vi "S2C_InitTest.vi"(8 "Error In":errorcluster, 11 "TestName":string) -> (0 "Error Out":errorcluster)   [LabVIEW 2015]
doc: "Detects an error and calls the error case to process the error."
uses:
  XML/S2C_XML_Globals.vi
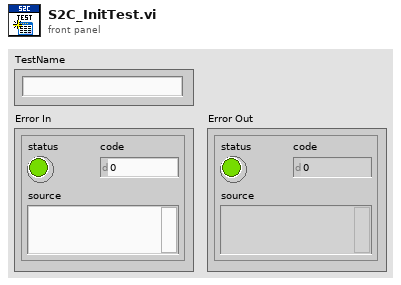
[diagram p1: front panel]
types:
  T1 = cluster{"TestName":string, "TestDateTime":string, "TestStatus":string, "Comment":string}
  T2 = cluster{"TestName":string, "TestDateTime":string, "TestStatus":string, "TestClientID":string, "IS_TestID":string, "TestMeta":string}
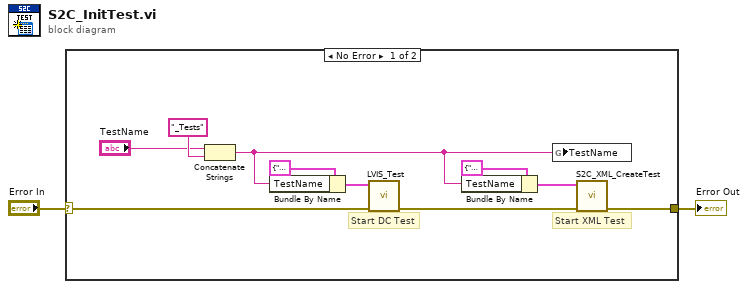
[diagram p0: block diagram]
diagram:
  n1 = case shown="No Error" "Error In" {
    selector: "Error In" -> [w4 w13]
    tunnel: [w8 w13] -> w1
    frame No Error {
      # "Start XML Test"
      # "Start DC Test"
      n2 = Concatenate Strings("TestName", "_Tests" ("string")) -> (w7:string)
      n3 = Bundle By Name(cluster=T2 {"TestName"="", "TestDateTime"="", "TestStatus"="", "TestClientID"="", "IS_TestID"="", "TestMeta"=""} ("TestInfo"), "TestName"=w7) -> (w11:T2)
      n4 = call "LVIS_Test.vi"("Error In"=w4, "TestInfo"=w11) -> ("Error Out"=w9:errorcluster)  [unwired: 9 in]
      n5 = Bundle By Name(cluster=T1 {"TestName"="", "TestDateTime"="", "TestStatus"="", "Comment"=""} ("TestData"), "TestName"=w7) -> (w5:T1)
      n6 = global write "S2C_XML_Globals.vi" "TestName"(w7) -> ()
      n7 = call "S2C_XML_CreateTest.vi"("Error In"=w9, "TestData"=w5) -> ("Error Out"=w8:errorcluster)  [unwired: 9 in]
    }
    frame Error {
    }
  }
  "Error Out" <- w1
